vi "Init Path.vi"(11 "Cave System In":T2) -> (1 "Start":i32, 2 "Path":T1, 3 "Cave System":T2)   [LabVIEW 2020]
uses:
  Path.ctl
  Cave.ctl
  Cave System.ctl
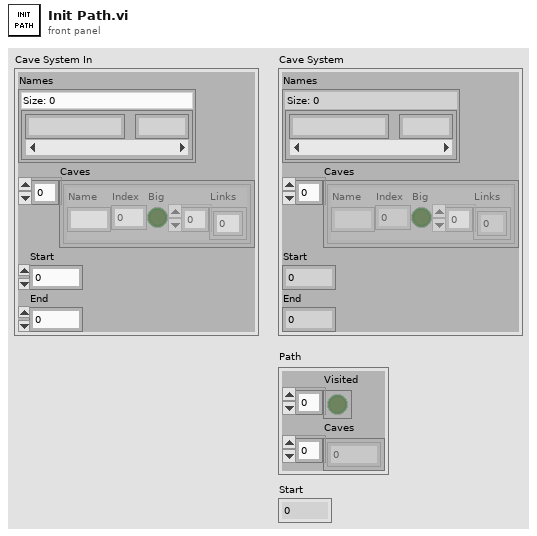
[diagram p1: front panel]
types:
  T1 = typedef "Path.ctl" = cluster{"Visited":bool[], "Caves":i32[]}
  T2 = typedef "Cave System.ctl" = cluster{"Names":map{string, i32}, "Caves":T3[], "Start":i32, "End":i32}
  T3 = typedef "Cave.ctl" = cluster{"Name":string, "Index":i32, "Big":bool, "Links":i32[]}
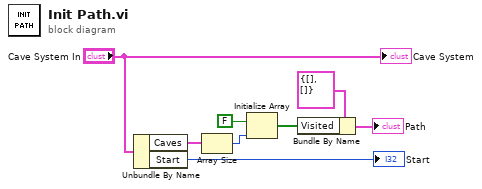
[diagram p0: block diagram]
diagram:
  n1 = Unbundle By Name("Cave System In") -> ("Caves"=w6:T3[], "Start"=→"Start":i32)
  n2 = Array Size(array=w6) -> (size(s)=w5:i32)
  n3 = Initialize Array(FALSE, w5) -> (w1:bool[])
  n4 = Bundle By Name(cluster=T1 {"Visited"=[], "Caves"=[]} ("Path"), "Visited"=w1) -> (→"Path":T1)
  "Cave System" <- "Cave System In"
